vi "RT Host - SvT discretise trajectory.vi"(5 "Which speed profile?":T4, 6 "Assistance Definition":T1={"Assistance Options"={"Assist Towards Target?"=FALSE, "Assist Ratchet?"=FALSE, "Form of Control?"=enum."Baseline", "Which Speed Profile?"=enum."Forward Skew"}, "Assistance Settings"={"Max Valley Width (mm)"=0.0, "Valley Width @ Tn (0-0.5)"=0.0, "Valley Width @ Tn-1 (0.5-1)"=0.0, "Valley Depth (0-1)"=0.0, "Stiffness (0-1)"=0.0, "Max Step Increment (mm)"=0.0, "Speed (0-1)"=0.0}}, 7 "Current Joy Global W/S Pos (mm)":dbl[](array[numeric])=[0.0, -90.0], 8 "error in":errorcluster, 9 "Target Global W/S Pos (mm)":dbl[](array[numeric])=[0.0, -90.0], 10 "Previous Target Global W/S Pos (mm)":dbl[](array[numeric])=[0.0, -90.0], 11 "New Target?":bool) -> (0 "error out":errorcluster, 1 "Speed Assistance?":bool, 2 "Global Ydes (mm)":dbl, 3 "Global Xdes (mm)":dbl, 4 "Reached Target?":bool)   [LabVIEW 2017]
doc: "This subVI discretises a trajectory path between the previous target position to the new one. The step increment is controlled by a normalised profile."
uses:
  Controls/hCAAR - speed profile.ctl
  Controls/RT Host - assistance definition.ctl
  Controls/RT Host - assistance options.ctl
  Controls/RT Host - form of control.ctl
  Controls/RT Host - assistance settings.ctl
panel:
  # "Inputs"
  # "Outputs"
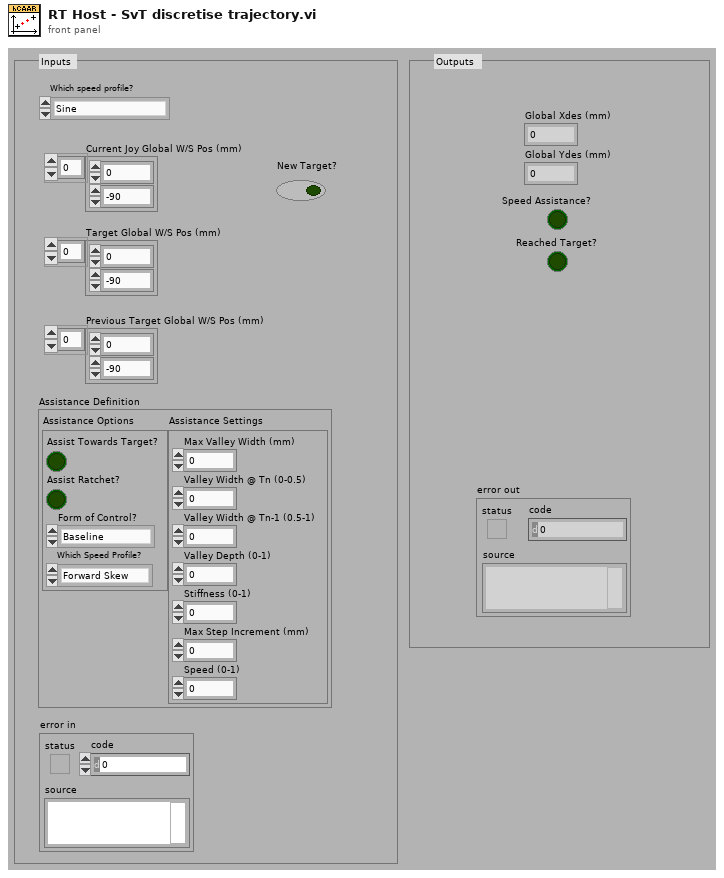
[diagram p1: front panel]
types:
  T1 = typedef "RT Host - assistance definition.ctl" = cluster{"Assistance Options":T2, "Assistance Settings":T5}
  T2 = typedef "RT Host - assistance options.ctl" = cluster{"Assist Towards Target?":bool, "Assist Ratchet?":bool, "Form of Control?":T3, "Which Speed Profile?":T4}
  T3 = typedef "RT Host - form of control.ctl" = enum16{"Baseline", "Gen II", "No Assist"}
  T4 = typedef "hCAAR - speed profile.ctl" = enum16{"Sine", "Sine With Initial Shunt", "Triangle", "Square", "Sawtooth", "Forward Skew", "User Defined"}
  T5 = typedef "RT Host - assistance settings.ctl" = cluster{"Max Valley Width (mm)":dbl, "Valley Width @ Tn (0-0.5)":dbl, "Valley Width @ Tn-1 (0.5-1)":dbl, "Valley Depth (0-1)":dbl, "Stiffness (0-1)":dbl, "Max Step Increment (mm)":dbl, "Speed (0-1)":dbl}
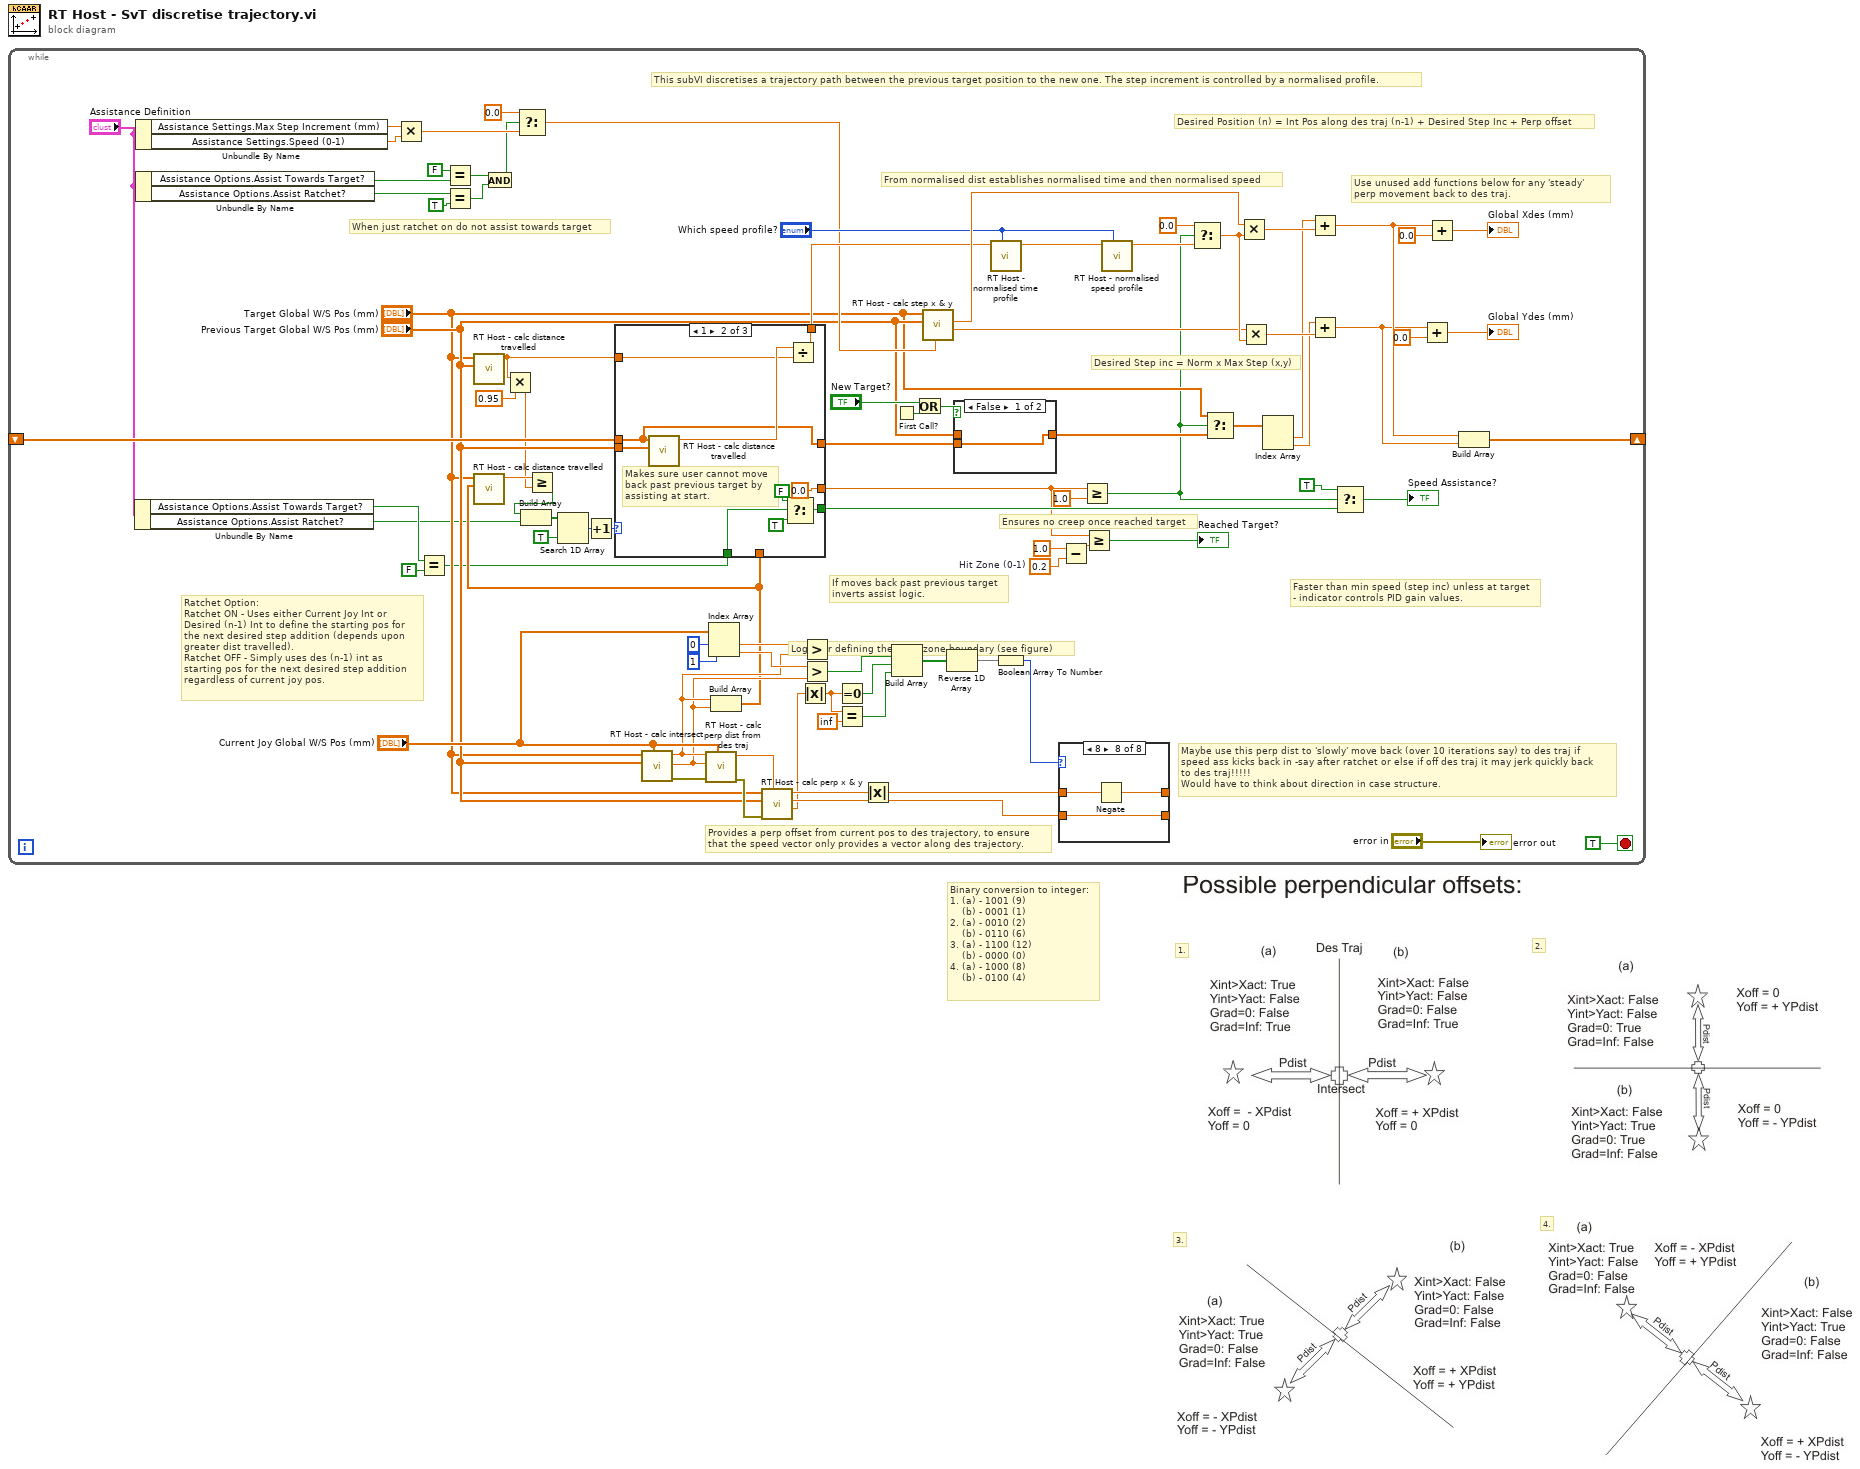
[diagram p0: block diagram]
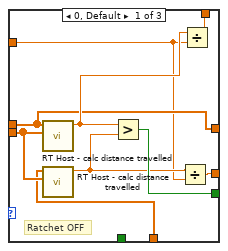
[diagram p2: hidden frame]
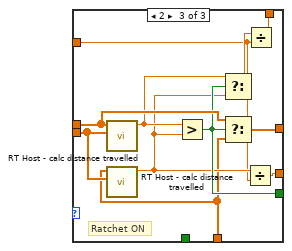
[diagram p3: hidden frame]
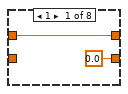
[diagram p4: hidden frame]
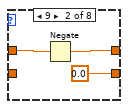
[diagram p5: hidden frame]
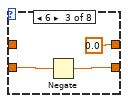
[diagram p6: hidden frame]
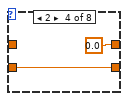
[diagram p7: hidden frame]
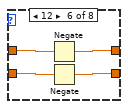
[diagram p9: hidden frame]
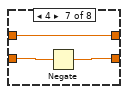
[diagram p10: hidden frame]
diagram:
  # "4."
  # "3."
  # "2."
  # "1."
  # "Binary conversion to integer:\n1. (a) - 1001 (9)\n    (b) - 0001 (1)\n2. (a) - 0010 (2)\n    (b) - 0110 (6)\n3. (a) - 1100 (12)\n    (b) - 0000 (0)\n4. (a) - 1000 (8)\n    (b) - 0100 (4)"
  n1 = while {
    shift-right: [w80] -> _
    shift-left: _ -> [w74]
    stop <- TRUE stop-if-true
    w12 = 0.2  # Hit Zone (0-1)
    # "If moves back past previous target\ninverts assist logic."
    # "When just ratchet on do not assist towards target"
    # "Maybe use this perp dist to 'slowly' move back (over 10 iterations say) to des traj if\nspeed ass kicks back in -say after ratchet or else if off des traj it may jerk quickly back\nto des traj!!!!!\nWould have to think about direction in case structure."
    # "Use unused add functions below for any 'steady' \nperp movement back to des traj."
    # "Desired Position (n) = Int Pos along des traj (n-1) + Desired Step Inc + Perp offset"
    # "Provides a perp offset from current pos to des trajectory, to ensure\nthat the speed vector only provides a vector along des trajectory."
    # "Logic for defining the dead zone boundary (see figure)"
    # "Faster than min speed (step inc) unless at target\n- indicator controls PID gain values."
    # "From normalised dist establishes normalised time and then normalised speed"
    # "Ratchet Option:\nRatchet ON - Uses either Current Joy Int or\nDesired (n-1) Int to define the starting pos for\nthe next desired step addition (depends upon\ngreater dist travelled).\nRatchet OFF - Simply uses des (n-1) int as\nstarting pos for the next desired step addition\nregardless of current joy pos."
    # "Ensures no creep once reached target"
    # "Desired Step inc = Norm x Max Step (x,y)"
    # "This subVI discretises a trajectory path between the previous target position to the new one. The step increment is controlled by a normalised profile."
    n2 = Unbundle By Name("Assistance Definition") -> ("Assistance Options.Assist Towards Target?"=w4:bool, "Assistance Options.Assist Ratchet?"=w3:bool)
    n3 = Unbundle By Name("Assistance Definition") -> ("Assistance Settings.Max Step Increment (mm)"=w9:dbl, "Assistance Settings.Speed (0-1)"=w8:dbl)
    n4 = Unbundle By Name("Assistance Definition") -> ("Assistance Options.Assist Towards Target?"=w6:bool, "Assistance Options.Assist Ratchet?"=w5:bool)
    n5 = Multiply(x=w9, y=w8) -> (x*y=w7:dbl)
    n6 = Equal?(x=w4, y=FALSE ("x")) -> (x = y?=w16:bool)
    n7 = Equal?(x=FALSE, y=w6) -> (x = y?=w2:bool)
    n8 = Equal?(x=w5, y=TRUE) -> (x = y?=w33:bool)
    n9 = call "RT Host - calc distance travelled.vi"("Origin Global W/S Pos (mm)"="Previous Target Global W/S Pos (mm)", "From Global W/S Pos (mm)"="Target Global W/S Pos (mm)") -> ("Distance Travelled"=w28:dbl)  [unwired: 8 in, 1 out]
    n10 = And(x=w2, y=w33) -> (x .and. y?=w1:bool)
    n11 = Multiply(x=w28, y=0.95) -> (x*y=w26:dbl)
    n12 = Select(t=0.0, s=w1, f=w7) -> (s? t:f=w32:dbl)
    n13 = call "RT Host - calc intersect.vi"("Current Position Global W/S Pos (mm)"="Current Joy Global W/S Pos (mm)", "Previous Target Global W/S Pos (mm)"="Previous Target Global W/S Pos (mm)", "Target Global W/S Pos (mm)"="Target Global W/S Pos (mm)") -> ("error out"=w65:errorcluster, "Global Yint (mm)"=w45:dbl, "Global Xint (mm)"=w46:dbl)  [unwired: 6 in]
    n14 = call "RT Host - calc perp dist from des traj.vi"("Current Global W/S Pos (mm)"="Current Joy Global W/S Pos (mm)", "error in (no error)"=w65, "Yint Global W/S (mm)"=w45, "Xint Global W/S (mm)"=w46) -> ("error out"=w64:errorcluster, "Perp Dist Global W/S (mm)"=w63:dbl)  [unwired: 6 in]
    n15 = Index Array(array="Current Joy Global W/S Pos (mm)", index #1=0 ("index"), index #2=1 ("index")) -> (element #1=w66:dbl, element #2=w67:dbl)
    n16 = Build Array(w46, w45) -> (w18:dbl[])
    n17 = call "RT Host - calc distance travelled.vi"("Origin Global W/S Pos (mm)"=w18, "From Global W/S Pos (mm)"="Target Global W/S Pos (mm)") -> ("Distance Travelled"=w29:dbl)  [unwired: 8 in, 1 out]
    n18 = Greater Or Equal?(x=w29, y=w26) -> (x >= y?=w25:bool)
    n19 = Build Array(w25, w3) -> (w24:bool[])
    n20 = Search 1D Array(1D array=w24, element=TRUE) -> (index of element=w22:i32)  [unwired: 1 in]
    n21 = Increment(x=w22) -> (x+1=w21:i32)
    n22 = case shown="1" w21 {
      tunnel: w74 -> [w96 w106 w120]
      tunnel: [w96 w106 w119] -> w73
      tunnel: [w95 w103 w114] -> w20
      tunnel: w18 -> [w92 _ w111]
      tunnel: "Previous Target Global W/S Pos (mm)" -> [w99 w109 w117]
      tunnel: [w98 w108 w115] -> w40
      tunnel: [w93 0.0 w112] -> w15
      tunnel: w28 -> [w91 w105 w110]
      tunnel: w16 -> [_ w101 _]
      frame 0, Default {
        # "Ratchet OFF"
        n23 = call "RT Host - calc distance travelled.vi"("Origin Global W/S Pos (mm)"=w99, "From Global W/S Pos (mm)"=w96) -> ("Distance Travelled"=w97:dbl)  [unwired: 8 in, 1 out]
        n24 = call "RT Host - calc distance travelled.vi"("Origin Global W/S Pos (mm)"=w99, "From Global W/S Pos (mm)"=w92) -> ("Distance Travelled"=w94:dbl)  [unwired: 8 in, 1 out]
        n25 = Greater?(x=w97, y=w94) -> (0:w95:bool)
        n26 = Divide(x=w94, y=w91) -> (x/y=w93:dbl)
        n27 = Divide(x=w97, y=w91) -> (x/y=w98:dbl)
      }
      frame 1 {
        # "Makes sure user cannot move\nback past previous target by\nassisting at start."
        n28 = call "RT Host - calc distance travelled.vi"("Origin Global W/S Pos (mm)"=w109, "From Global W/S Pos (mm)"=w106) -> ("Distance Travelled"=w107:dbl)  [unwired: 8 in, 1 out]
        n29 = Select(t=FALSE, s=w101, f=TRUE) -> (s? t:f=w103:bool)
        n30 = Divide(x=w107, y=w105) -> (x/y=w108:dbl)
      }
      frame 2 {
        # "Ratchet ON"
        n31 = call "RT Host - calc distance travelled.vi"("Origin Global W/S Pos (mm)"=w117, "From Global W/S Pos (mm)"=w120) -> ("Distance Travelled"=w118:dbl)  [unwired: 8 in, 1 out]
        n32 = call "RT Host - calc distance travelled.vi"("Origin Global W/S Pos (mm)"=w117, "From Global W/S Pos (mm)"=w111) -> ("Distance Travelled"=w113:dbl)  [unwired: 8 in, 1 out]
        n33 = Greater?(x=w118, y=w113) -> (0:w114:bool)
        n34 = Select(t=w118, s=w114, f=w113) -> (s? t:f=w116:dbl)
        n35 = Select(t=w120, s=w114, f=w111) -> (s? t:f=w119:dbl[])
        n36 = Divide(x=w113, y=w110) -> (x/y=w112:dbl)
        n37 = Divide(x=w116, y=w110) -> (x/y=w115:dbl)
      }
    }
    n38 = call "RT Host - calc perp x & y.vi"("Perp Dist Global W/S (mm)"=w63, "error in (no error)"=w64, "Previous Target Global W/S Pos (mm)"="Previous Target Global W/S Pos (mm)", "Target Global W/S Pos (mm)"="Target Global W/S Pos (mm)") -> ("Gradient"=w52:dbl, "Perp Y Adjustment (mm)"=w62:dbl, "Perp X Adjustment (mm)"=w59:dbl)  [unwired: 4 in, 1 out]
    n39 = Absolute Value(x=w52) -> (abs(x)=w51:dbl)
    n40 = Greater?(x=w66, y=w46) -> (0:w55:bool)
    n41 = Greater?(x=w67, y=w45) -> (0:w56:bool)
    n42 = Equal To 0?(x=w51) -> (x = 0?=w57:bool)
    n43 = Equal?(x=w51, y=inf) -> (x = y?=w53:bool)
    n44 = Absolute Value(x=w59) -> (abs(x)=w58:dbl)
    n45 = First Call?() -> (First Call?: T/F=w75:bool)
    n46 = Build Array(w55, w56, w57, w53) -> (w50:bool[])
    n47 = Or(x="New Target?", y=w75) -> (x .or. y?=w77:bool)
    n48 = call "RT Host - calc step x & y.vi"("Max Step Inc (mm)"=w32, "Previous Target Global W/S Pos (mm)"="Previous Target Global W/S Pos (mm)", "Target Global W/S Pos (mm)"="Target Global W/S Pos (mm)") -> ("Max Y Increment (mm)"=w83:dbl, "Max X Increment (mm)"=w84:dbl)  [unwired: 6 in, 1 out]
    n49 = Reverse 1D Array(array=w50) -> (reversed array=w48:bool[])
    n50 = case shown="False" w77 {
      tunnel: "Previous Target Global W/S Pos (mm)" -> [_ w144]
      tunnel: [w143 w144] -> w68
      tunnel: w73 -> [w143 _]
      frame False {
      }
      frame True {
      }
    }
    n51 = call "RT Host - normalised time profile.vi"("Which speed profile?"="Which speed profile?", "X Input (normalised 0-1)"=w40) -> ("Y output (normalised 0-1)"=w39:dbl)  [unwired: 7 in, 2 out]
    n52 = Boolean Array To Number(Boolean array=w48) -> (number=w49:u32)
    n53 = case shown="8" w49 {
      tunnel: w58 -> [w122 w125 _ _ w132 w136 w139 w142]
      tunnel: w62 -> [_ _ w128 w130 w131 w135 w138 w141]
      tunnel: [w122 w124 0.0 0.0 w132 w134 w139 w140] -> _
      tunnel: [0.0 ("-x") 0.0 ("-x") w126 w130 w131 w133 w137 w141] -> _
      frame 1 {
      }
      frame 9 {
        n54 = Negate(x=w125) -> (-x=w124:dbl)
      }
      frame 6 {
        n55 = Negate(x=w128) -> (-x=w126:dbl)
      }
      frame 2 {
      }
      frame 0, Default {
      }
      frame 12 {
        n56 = Negate(x=w136) -> (-x=w134:dbl)
        n57 = Negate(x=w135) -> (-x=w133:dbl)
      }
      frame 4 {
        n58 = Negate(x=w138) -> (-x=w137:dbl)
      }
      frame 8 {
        n59 = Negate(x=w142) -> (-x=w140:dbl)
      }
    }
    n60 = Subtract(x=1.0 ("y"), y=w12) -> (x-y=w10:dbl)
    n61 = Greater Or Equal?(x=w15, y=1.0) -> (x >= y?=w14:bool)
    n62 = Greater Or Equal?(x=w15, y=w10) -> (x >= y?=→"Reached Target?":bool)
    n63 = call "RT Host - normalised speed profile.vi"("Which speed profile?"="Which speed profile?", "X input (normalised 0-1)"=w39) -> ("Y output (normalised 0-1)"=w71:dbl)  [unwired: 7 in, 2 out]
    n64 = Select(t=0.0, s=w14, f=w71) -> (s? t:f=w86:dbl)
    n65 = Select(t="Target Global W/S Pos (mm)", s=w14, f=w68) -> (s? t:f=w69:dbl[])
    n66 = Multiply(x=w84, y=w86) -> (x*y=w90:dbl)
    n67 = Multiply(x=w83, y=w86) -> (x*y=w89:dbl)
    n68 = Index Array(array=w69) -> (element #1=w79:dbl, element #2=w78:dbl)  [unwired: 2 in]
    n69 = Add(x=w79, y=w90) -> (x+y=w82:dbl)
    n70 = Add(x=w78, y=w89) -> (x+y=w81:dbl)
    n71 = Select(t=TRUE, s=w14, f=w20) -> (s? t:f=→"Speed Assistance?":bool)
    n72 = Add(x=w81, y=0.0) -> (x+y=→"Global Ydes (mm)":dbl)
    n73 = Add(x=w82, y=0.0) -> (x+y=→"Global Xdes (mm)":dbl)
    n74 = Build Array(w82, w81) -> (w80:dbl[])
    "error out" <- "error in"
  }
